vi "resetProfileStepCounter.vi"(8 "error in (no error)":errorcluster, 11 "Model in":refnum<class "Model.lvclass">) -> (0 "error out":errorcluster, 3 "Model out":refnum<class "Model.lvclass">)   [LabVIEW 2013, in "Model.lvclass"]
uses:
  Model.lvclass
  Model.lvclass/Model.ctl
  ApplicationElements/Log/TestDataLog/TestDataLog.lvclass/TestDataLog.ctl
  UserEvents/UserEvents.lvclass/UserEvents.ctl
  ApplicationElements/TestMonitor/TestMonitor.lvclass/TestMonitor.ctl
  ApplicationElements/TestMonitor/TestMonitor.lvclass
  UserEvents/UserEvents.lvclass
  ApplicationElements/Log/TestDataLog/TestDataLog.lvclass
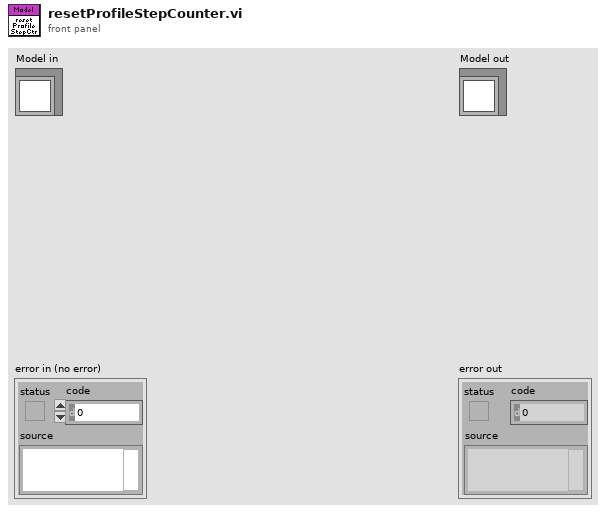
[diagram p1: front panel]
types:
  T1 = typedef "AITDTTypedefs.lvlib/PubDataEvents.ctl" = cluster{"State":refnum<user-event>, "ErrorCode":refnum<user-event>, "OutputData":refnum<user-event>, "InputData":refnum<user-event>, "TestStatus":refnum<user-event>, "LogPath":refnum<user-event>, "TemperatureSetpointRequest":refnum<user-event>, "TemperatureSettling":refnum<user-event>}
  T2 = typedef "TestParameters.ctl" = cluster{"Number of cycles for complete test":u32, "Cycle profile":T3, "PGA Gain Coefficients":u8[], "Temperature Transition Wait Time":dbl[unit], "Temperature Settled StDev":dbl[unit], "Temperature Settling Sample Size":u16, "Bridge Measurement Sample Size":u16}
  T3 = typedef "CycleProfileConfig.ctl" = cluster{"Temperature Setpoint":dbl[unit][], "Soak Time":dbl[unit][], "Gain Stabilization Time":dbl[unit][], "Pause After Step":dbl[unit][]}
  T4 = typedef "AITDTTypedefs.lvlib/TestStatus.ctl" = cluster{"activeCycle":u32, "activeProfileStep":u32, "demandedCycles":u32, "demandedProfileSteps":u32, "temperatureSetpoint":dbl[unit], "pgaGainCoefficient":u16}
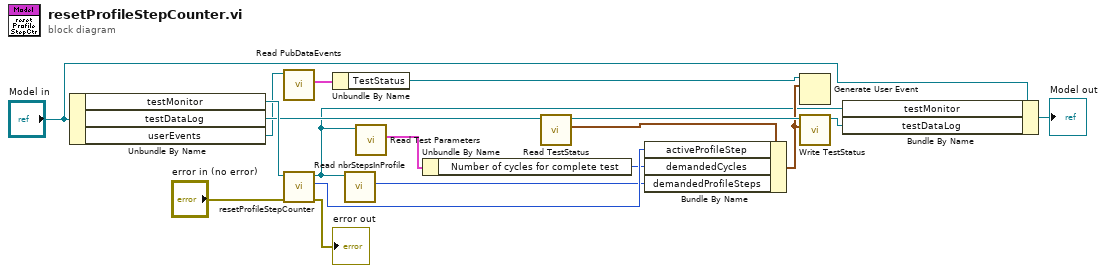
[diagram p0: block diagram]
diagram:
  n1 = Unbundle By Name("Model in") -> ("testMonitor"=w18:refnum<class "TestMonitor.lvclass">, "testDataLog"=w12:refnum<class "TestDataLog.lvclass">, "userEvents"=w5:refnum<class "UserEvents.lvclass">)
  n2 = call "Read PubDataEvents.vi"("UserEvents in"=w5) -> ("PubDataEvents"=w7:T1)  [unwired: 9 in, 1 out]
  n3 = call "resetProfileStepCounter.vi"("error in (no error)"="error in (no error)", "TestMonitor in"=w18) -> ("error out"=→"error out":errorcluster, "activeProfileStep"=w9:u32, "TestMonitor out"=w1:refnum<class "TestMonitor.lvclass">)  [unwired: 7 in]
  n4 = Unbundle By Name(w7) -> ("TestStatus"=w6:refnum<user-event>)
  n5 = call "Read nbrStepsInProfile.vi"("TestMonitor in"=w1) -> ("nbrStepsInProfile"=w2:u32)  [unwired: 9 in, 1 out]
  n6 = call "Read Test Parameters.vi"("TestMonitor in"=w1) -> ("Test Parameters"=w4:T2)  [unwired: 9 in, 1 out]
  n7 = Unbundle By Name(w4) -> ("Number of cycles for complete test"=w3:u32)
  n8 = call "Read TestStatus.vi"("Logger in"=w12) -> ("TestStatus"=w13:T4, "Logger out"=w11:refnum<class "TestDataLog.lvclass">)  [unwired: 9 in]
  n9 = Bundle By Name(cluster=w13, "activeProfileStep"=w9, "demandedCycles"=w3, "demandedProfileSteps"=w2) -> (w8:T4)
  n10 = Generate User Event(user event=w6, event data cluster=w8) -> ()  [unwired: 2 in, 2 out]
  n11 = call "Write TestStatus.vi"("TestStatus"=w8, "Logger in"=w11) -> ("Logger out"=w10:refnum<class "TestDataLog.lvclass">)  [unwired: 9 in]
  n12 = Bundle By Name(cluster="Model in", "testMonitor"=w1, "testDataLog"=w10) -> (→"Model out":refnum<class "Model.lvclass">)
